vi "Auto 10.vi"(8 "Error In":errorcluster) -> (0 "Error Out":errorcluster)   [LabVIEW 2014]
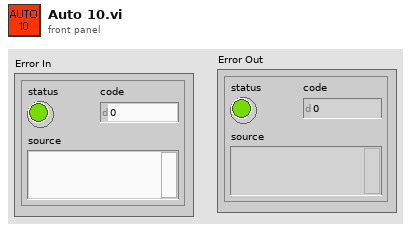
[diagram p1: front panel]
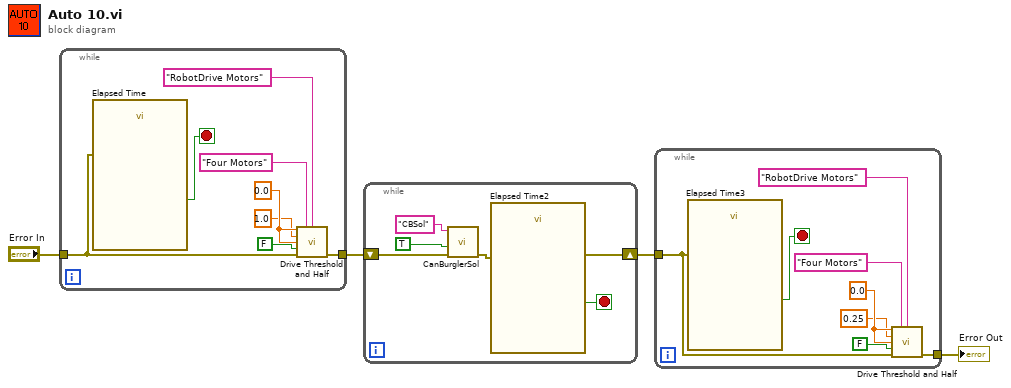
[diagram p0: block diagram]
diagram:
  n1 = while {
    tunnel: [w9] -> w4
    tunnel: "Error In" -> [w6]
    stop <- w7 stop-if-true
    w8 = 0.0 ("Arm Value")
    n2 = call "Elapsed Time"("error in (no error)"=w6) -> ("Time has Elapsed"=w7:bool)  [unwired: 11 in, 7 out]
    n3 = call "Drive Threshold and Half.vi"("X In"=w8, "Drive refnum name"="Four Motors" ("refnum name"), "Send to DB Name"="RobotDrive Motors" ("Name"), "Y In"=1.0 ("X In"), "R In"=w8, "Speed Toggle"=FALSE ("Grabber Open/Close"), "Error In"=w6) -> ("Error Out"=w9:errorcluster)  [unwired: 8 in]
  }
  n4 = while {
    shift-right: [w14] -> w3
    shift-left: w4 -> [w18]
    stop <- w13 stop-if-true
    n5 = call "CanBurglerSol.vi"("Error In"=w18, "Grabber Open/Close"=TRUE, "refnum name"="CBSol") -> ("Error Out"=w15:errorcluster)  [unwired: 8 in]
    n6 = call "Elapsed Time2"("error in (no error)"=w15) -> ("Time has Elapsed"=w13:bool, "error out"=w14:errorcluster)  [unwired: 11 in, 6 out]
  }
  n7 = while {
    tunnel: [w23] -> w1
    tunnel: w3 -> [w20]
    stop <- w21 stop-if-true
    w22 = 0.0 ("Arm Value")
    n8 = call "Elapsed Time3"("error in (no error)"=w20) -> ("Time has Elapsed"=w21:bool)  [unwired: 11 in, 7 out]
    n9 = call "Drive Threshold and Half.vi"("X In"=w22, "Drive refnum name"="Four Motors" ("refnum name"), "Send to DB Name"="RobotDrive Motors" ("Name"), "Y In"=0.25 ("X In"), "R In"=w22, "Speed Toggle"=FALSE ("Grabber Open/Close"), "Error In"=w20) -> ("Error Out"=w23:errorcluster)  [unwired: 8 in]
  }
  "Error Out" <- w1
